vi "Coord window-Clear coordinates list.vi"(8 "error in (no error)":errorcluster, 10 "Enabled? (T)":bool=TRUE) -> (0 "error out":errorcluster)   [LabVIEW 2013]
uses:
  Globals/Coord window-Globals.vi
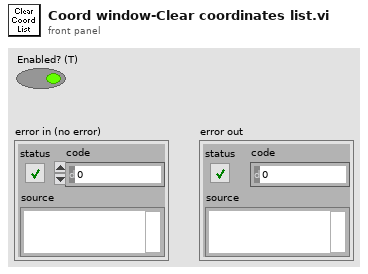
[diagram p1: front panel]
types:
  T1 = typedef "Coordinate list window refs.ctl" = cluster{"Window Name (i.e. Key)":string, "menu reference":refnum<k9>, "VI's reference":refnum<vi>, "Pane 1":refnum<vi>, "Pane 2":refnum<vi>, "Coord Listbox":refnum<vi>, "File name":refnum<vi>, "Picture Map":refnum<vi>, "Stage XYZ Position ind.":refnum<vi>}
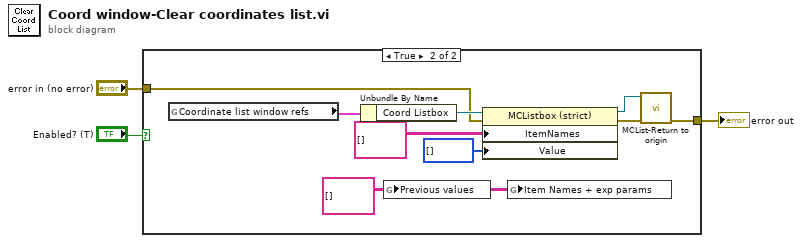
[diagram p0: block diagram]
diagram:
  n1 = case shown="True" "Enabled? (T)" {
    tunnel: "error in (no error)" -> [w4 w9]
    tunnel: [w4 w6] -> w2
    frame False {
    }
    frame True {
      w5 = string[][] [] ("Previous values")
      n2 = global read "Coord window-Globals.vi" "Coordinate list window refs"() -> (w10:T1)
      n3 = Unbundle By Name(w10) -> ("Coord Listbox"=w11:refnum<vi>)
      n4 = global write "Coord window-Globals.vi" "Previous values"(w5) -> ()
      n5 = property on="Property Node" class="MCListbox (strict)"(reference=w11, error in=w9, "ItemNames"=string[][] [] ("Item Names"), "Value"=i32[] []) -> (reference out=w8:refnum<vi>, error out=w7:errorcluster)
      n6 = global write "Coord window-Globals.vi" "Item Names + exp params"(w5) -> ()
      n7 = call "MCList-Return to origin.vi"("error in (no error)"=w7, "MulticolumnListbox in"=w8) -> ("error out"=w6:errorcluster)  [unwired: 8 in, 1 out]
    }
  }
  "error out" <- w2
